vi "fetchBTFData_chaos.vi"(0 "Funcion":u16(ring) items=["Init", "Run", "Close"], 1 "!CHAOS WAN url":u32=10000) -> (3 "lastTrigger":i32, 4 "Array":i32[](array[numeric]), 6 "ReadError":bool, 7 "DataReady":bool)   [LabVIEW 2014]
panel:
  # "Version:\n- 1.0 UDP to MC\n- 1.1 deduce dataready \n\nto be done:\n- manage errori"
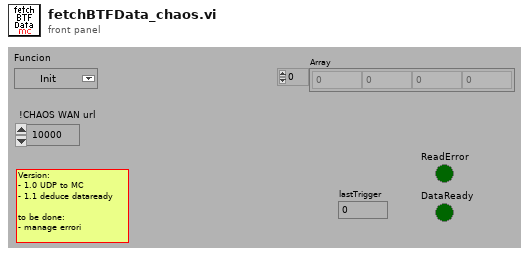
[diagram p1: front panel]
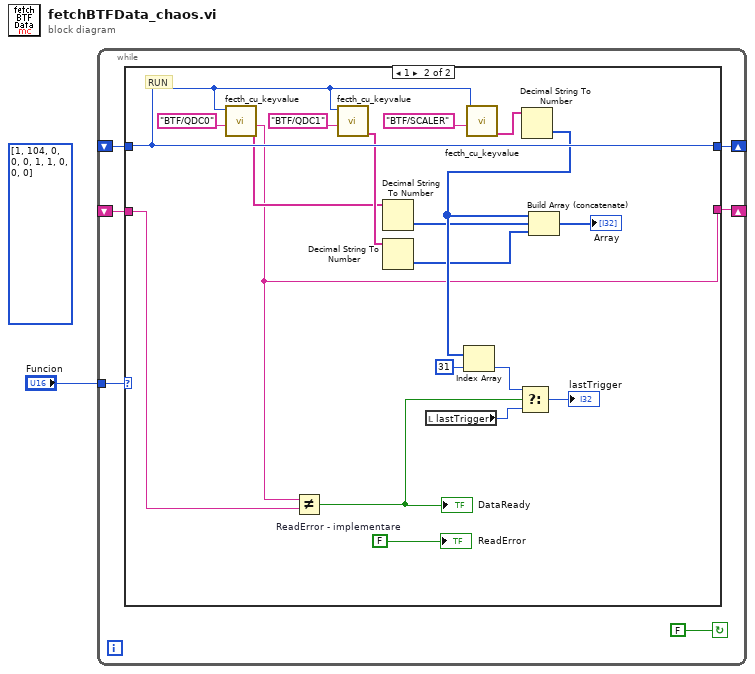
[diagram p0: block diagram]
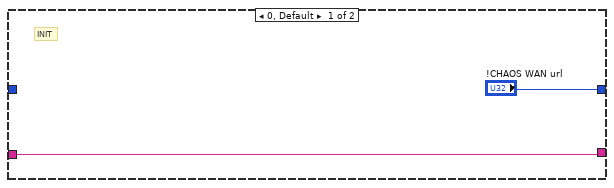
[diagram p2: hidden frame]
diagram:
  (unwired) i32[] [1, 104, 0, 0, 0, 1, 1, 0, 0, 0]
  n1 = while {
    shift-left: _ -> [w6]
    shift-right: [w5] -> _
    tunnel: "Funcion" -> [w7]
    shift-right: [w3] -> _
    shift-left: _ -> [w2]
    stop <- FALSE continue-if-true
    n2 = case shown="1" w7 {
      tunnel: w6 -> [_ w19]
      tunnel: ["!CHAOS WAN url" w19] -> w5
      tunnel: [w8 w10] -> w3
      tunnel: w2 -> [w8 w25]
      frame 0, Default {
        # "INIT"
      }
      frame 1 {
        w23 = FALSE  # ReadError - implementare
        # "RUN"
        n3 = call "fecth_cu_keyvalue.vi"("cuname"="BTF/QDC0", "handleConnection"=w19) -> ("data out"=w13:string[], "timestemp"=w10:string)  [unwired: 4 in, 4 out]
        n4 = Not Equal?(x=w10, y=w25) -> (x != y?=w24:bool)
        "DataReady" <- w24
        n5 = call "fecth_cu_keyvalue.vi"("cuname"="BTF/QDC1", "handleConnection"=w19) -> ("data out"=w14:string[])  [unwired: 4 in, 5 out]
        n6 = Decimal String To Number(string=w13) -> (number=w12:i32[])  [unwired: 2 in, 1 out]
        n7 = Decimal String To Number(string=w14) -> (number=w11:i32[])  [unwired: 2 in, 1 out]
        n8 = local read "lastTrigger"() -> (w26:i32)
        n9 = call "fecth_cu_keyvalue.vi"("cuname"="BTF/SCALER", "handleConnection"=w19) -> ("data out"=w17:string[])  [unwired: 4 in, 5 out]
        n10 = Decimal String To Number(string=w17) -> (number=w16:i32[])  [unwired: 2 in, 1 out]
        n11 = Index Array(array=w16, index=31) -> (element=w27:i32)
        n12 = Select(t=w27, s=w24, f=w26) -> (s? t:f=→"lastTrigger":i32)
        n13 = Build Array (concatenate)(w16, w12, w11) -> (→"Array":i32[])
        "ReadError" <- w23
      }
    }
  }
